vi "Coppia minima.vi"() -> ()   [LabVIEW 2016]
panel:
  in  "%Coppia minima":dbl
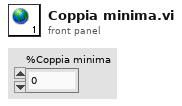
[diagram p1: front panel]
diagram:
